vi "counter_monitor.vi"() -> ()   [LabVIEW 2013]
uses:
  <vilib>/DAQmx/read.llb/DAQmx Read (Counter DBL 1Chan 1Samp).vi
  <vilib>/DAQmx/miscellaneous.llb/DAQmx Fill In Error Info.vi
panel:
  in  "Y":dbl format="%#_13g"
  in  "X":dbl format="%#_13g"
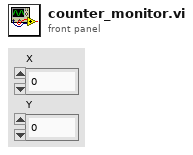
[diagram p1: front panel]
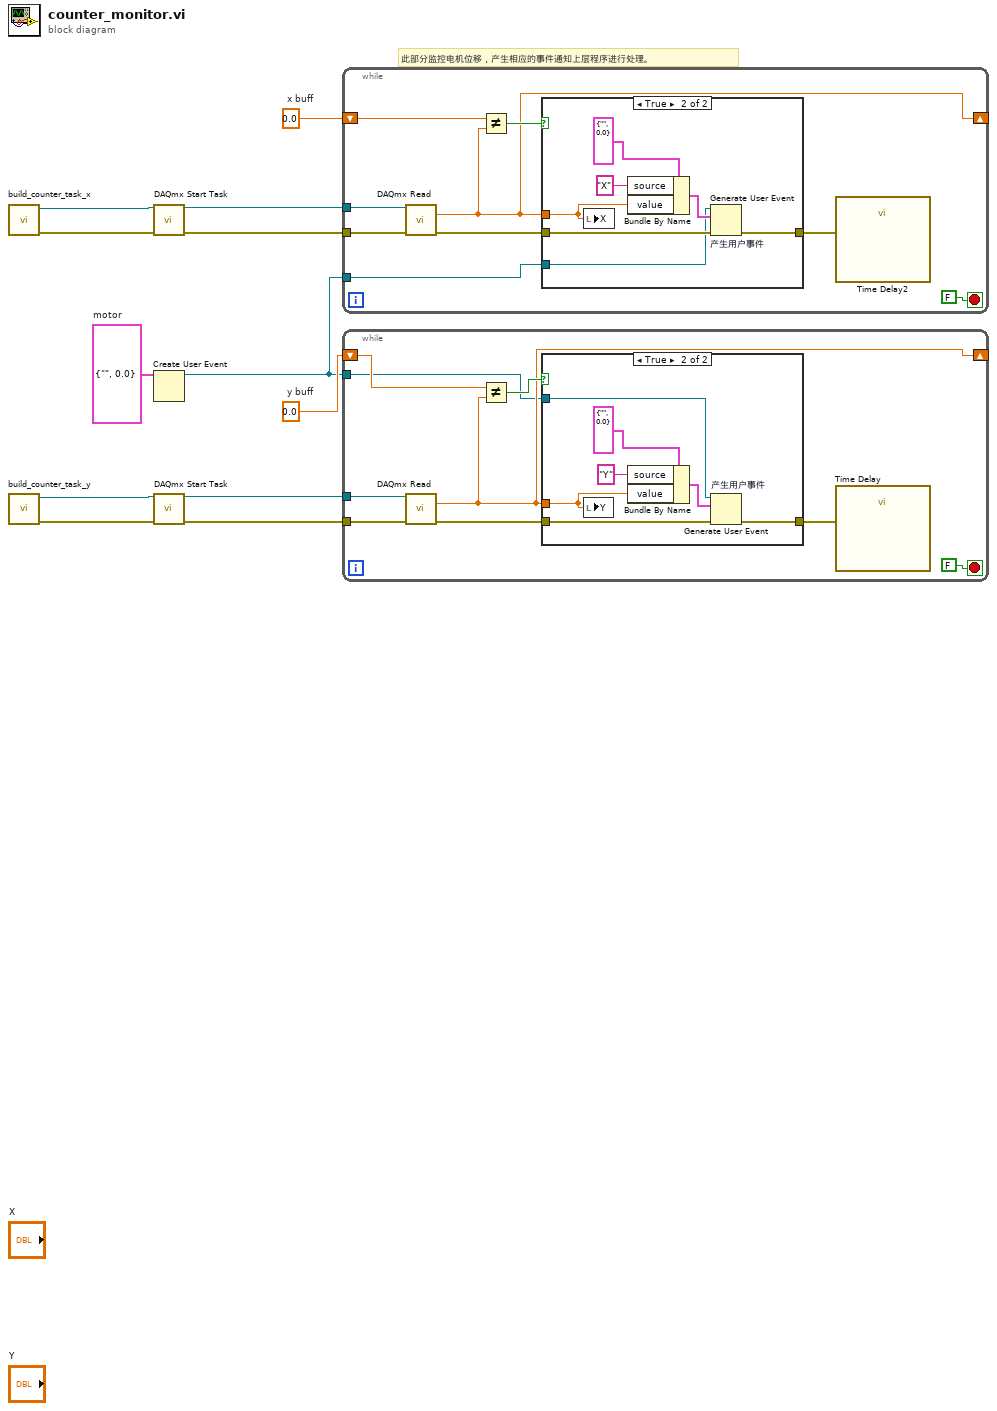
[diagram p0: block diagram]
diagram:
  w2 = cluster{"source":string, "value":dbl} {"source"="", "value"=0.0}  # motor
  w7 = 0.0  # x buff
  w10 = 0.0  # y buff
  # "此部分监控电机位移，产生相应的事件通知上层程序进行处理。"
  n1 = call "build_counter_task_x.vi"() -> ("error out"=w6:errorcluster, "task out"=w5:refnum<k21>)  [unwired: 10 in]
  n2 = call "build_counter_task_y.vi"() -> ("error out"=w3:errorcluster, "task out"=w4:refnum<k21>)  [unwired: 10 in]
  n3 = call <vilib>:"DAQmx Start Task.vi"("task/channels in"=w5, "error in"=w6) -> ("task out"=w9:refnum<k21>, "error out"=w8:errorcluster)  [unwired: 12 in]
  n4 = Create User Event(user event datatype=w2) -> (user event=w1:refnum<user-event>)  [unwired: 1 in, 1 out]
  n5 = call <vilib>:"DAQmx Start Task.vi"("task/channels in"=w4, "error in"=w3) -> ("task out"=w12:refnum<k21>, "error out"=w11:errorcluster)  [unwired: 12 in]
  n6 = while {
    tunnel: w9 -> [w19]
    tunnel: w8 -> [w21]
    shift-right: [w17] -> _
    shift-left: w7 -> [w20]
    tunnel: w1 -> [w13]
    stop <- FALSE stop-if-true
    n7 = call-poly <vilib>:"DAQmx Read.vi"("task/channels in"=w19, "error in"=w21) -> ("data"=w17:dbl, "error out"=w16:errorcluster)  [unwired: 11 in, 1 out]
    n8 = Not Equal?(x=w20, y=w17) -> (x != y?=w18:bool)
    n9 = case shown="True" w18 {
      tunnel: w17 -> [_ w23]
      tunnel: w16 -> [w22 w26]
      tunnel: [w22 w25] -> w14
      tunnel: w13 -> [_ w24]
      frame False {
      }
      frame True {
        n10 = local write "X"(w23) -> ()
        n11 = Bundle By Name(cluster=cluster{"source":string, "value":dbl} {"source"="", "value"=0.0} ("事件数据"), "source"="X", "value"=w23) -> (w27:cluster{"source":string, "value":dbl})
        n12 = Generate User Event "产生用户事件"(user event=w24, event data cluster=w27, error in=w26) -> (error out=w25:errorcluster)  [unwired: 1 in, 1 out]
      }
    }
    n13 = call "Time Delay2"("error in (no error)"=w14) -> ()  [unwired: 10 in, 1 out]
  }
  n14 = while {
    tunnel: w12 -> [w36]
    tunnel: w11 -> [w38]
    shift-right: [w34] -> _
    shift-left: w10 -> [w37]
    tunnel: w1 -> [w30]
    stop <- FALSE stop-if-true
    n15 = call-poly <vilib>:"DAQmx Read.vi"("task/channels in"=w36, "error in"=w38) -> ("data"=w34:dbl, "error out"=w33:errorcluster)  [unwired: 11 in, 1 out]
    n16 = Not Equal?(x=w37, y=w34) -> (x != y?=w35:bool)
    n17 = case shown="True" w35 {
      tunnel: w34 -> [_ w40]
      tunnel: w33 -> [w39 w42]
      tunnel: [w39 w41] -> w31
      tunnel: w30 -> [_ w43]
      frame False {
      }
      frame True {
        n18 = local write "Y"(w40) -> ()
        n19 = Bundle By Name(cluster=cluster{"source":string, "value":dbl} {"source"="", "value"=0.0} ("事件数据"), "source"="Y", "value"=w40) -> (w44:cluster{"source":string, "value":dbl})
        n20 = Generate User Event "产生用户事件"(user event=w43, event data cluster=w44, error in=w42) -> (error out=w41:errorcluster)  [unwired: 1 in, 1 out]
      }
    }
    n21 = call "Time Delay"("error in (no error)"=w31) -> ()  [unwired: 10 in, 1 out]
  }
